vi "UT - Big Data.vi"(11 "Size":i32=1) -> (0 "error out":errorcluster)   [LabVIEW 2019]
uses:
  HDF5 Tools.lvlib
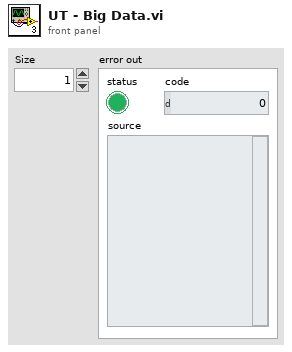
[diagram p1: front panel]
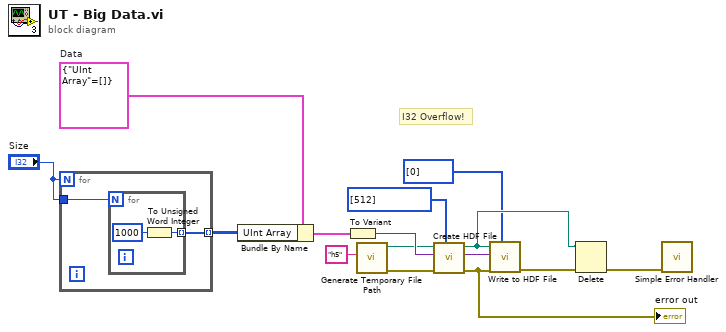
[diagram p0: block diagram]
diagram:
  w13 = cluster{"UInt Array":u16[][]} {"UInt Array"=[]}  # Data
  # "I32 Overflow!"
  n1 = for {
    N: "Size" -> [_]
    tunnel: [w17] -> w15 mode=indexing
    tunnel: "Size" -> [w16]
    n2 = for {
      N: w16 -> [_]
      tunnel: [w18] -> w17 mode=indexing
      n3 = To Unsigned Word Integer(number=1000) -> (unsigned 16bit integer=w18:u16)
    }
  }
  n4 = Bundle By Name(cluster=w13, "UInt Array"=w15) -> (w5:cluster{"UInt Array":u16[][]})
  n5 = To Variant(anything=w5) -> (Variant=w12:variant)
  n6 = call <vilib>:"Generate Temporary File Path.vi"("Temporary File Extension (tmp)"="h5") -> ("error out"=w11:errorcluster, "Unique Temporary File Path"=w10:path)  [unwired: 9 in]
  n7 = call "Create HDF File.vi"("Dims"=u64[] [512], "error in (no error)"=w11, "variant"=w12, "path"=w10) -> ("error out"=w2:errorcluster, "variant out"=w9:variant, "path out"=w7:path)  [unwired: 5 in]
  "error out" <- w2
  n8 = call "Write to HDF File.vi"("indices"=u64[] [0], "error in (no error)"=w2, "variant"=w9, "path"=w7) -> ("error out"=w8:errorcluster)  [unwired: 7 in]
  n9 = Delete(path (use dialog)=w7, error in=w8) -> (error out=w1:errorcluster)  [unwired: 3 in, 2 out]
  n10 = call <vilib>:"Simple Error Handler.vi"("error in (no error)"=w1) -> ()  [unwired: 4 in, 5 out]
